vi "Drive Handling.vi"(1 "Reverse":bool, 2 "Straight":bool, 3 "Low Sensitivity":bool, 4 "Z":dbl, 5 "Y":dbl, 6 "X":dbl) -> (0 "Axes Magnitudes":cluster{"X":dbl, "Y":dbl, "Z":dbl})   [LabVIEW 2017, in "Huskie Swerve.lvlib"]
uses:
  Huskie Swerve.lvlib
panel:
  in  "Low Sensitivity x & y":dbl=1.7 format="%#_13g"
  in  "Low Sensitivity z":dbl=1.9 format="%#_13g"
  in  "Default Sensitivity x & y":dbl=1.4 format="%#_13g"
  in  "Default Sensitivity z":dbl=1.6 format="%#_13g"
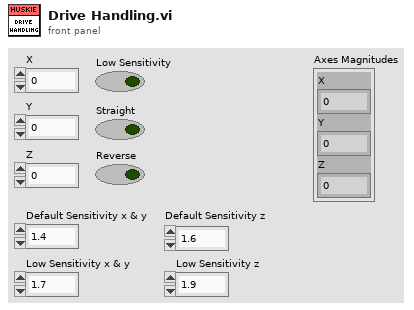
[diagram p1: front panel]
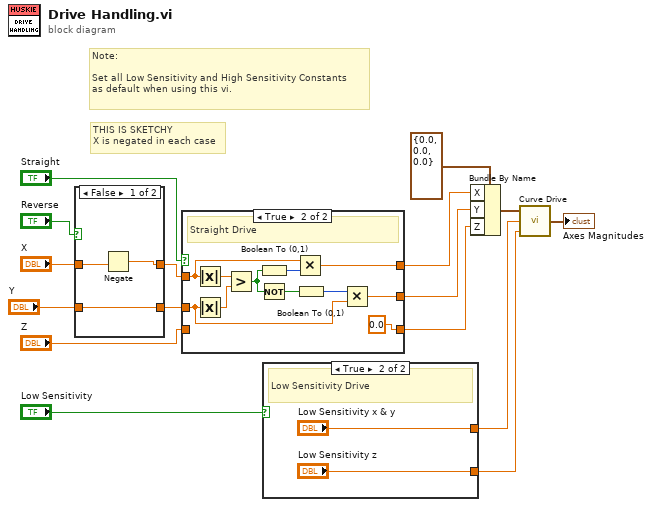
[diagram p0: block diagram]
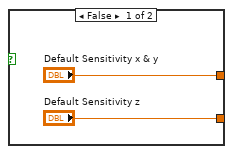
[diagram p2: hidden frame]
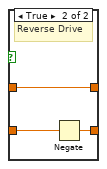
[diagram p4: hidden frame]
diagram:
  # "THIS IS SKETCHY\nX is negated in each case"
  # "Note: \n\nSet all Low Sensitivity and High Sensitivity Constants\nas default when using this vi."
  n1 = case shown="False" "Reverse" {
    tunnel: [w17 w20] -> w12
    tunnel: "X" -> [w18 w20]
    tunnel: [w19 w22] -> w13
    tunnel: "Y" -> [w19 w21]
    frame False {
      n2 = Negate(x=w18) -> (-x=w17:dbl)
    }
    frame True {
      # "Reverse Drive"
      n3 = Negate(x=w21) -> (-x=w22:dbl)
    }
  }
  n4 = case shown="True" "Straight" {
    tunnel: w12 -> [w25 w34]
    tunnel: w13 -> [w24 w29]
    tunnel: "Z" -> [w23 _]
    tunnel: [w25 w36] -> w5
    tunnel: [w23 0.0] -> w3
    tunnel: [w24 w35] -> w2
    frame False {
    }
    frame True {
      # "Straight Drive"
      n5 = Absolute Value(x=w34) -> (abs(x)=w28:dbl)
      n6 = Absolute Value(x=w29) -> (abs(x)=w27:dbl)
      n7 = Greater?(x=w28, y=w27) -> (0:w32:bool)
      n8 = Boolean To (0,1)(Boolean=w32) -> (0, 1=w33:i16)
      n9 = Not(x=w32) -> (.not. x?=w31:bool)
      n10 = Multiply(x=w34, y=w33) -> (x*y=w36:dbl)
      n11 = Boolean To (0,1)(Boolean=w31) -> (0, 1=w30:i16)
      n12 = Multiply(x=w30, y=w29) -> (x*y=w35:dbl)
    }
  }
  n13 = case shown="True" "Low Sensitivity" {
    tunnel: ["Default Sensitivity x & y" "Low Sensitivity x & y"] -> w8
    tunnel: ["Default Sensitivity z" "Low Sensitivity z"] -> w7
    frame False {
    }
    frame True {
      # "Low Sensitivity Drive"
    }
  }
  n14 = Bundle By Name(cluster=cluster{"X":dbl, "Y":dbl, "Z":dbl} {"X"=0.0, "Y"=0.0, "Z"=0.0} ("input cluster"), "X"=w5, "Y"=w2, "Z"=w3) -> (w4:cluster{"X":dbl, "Y":dbl, "Z":dbl})
  n15 = call "Curve Drive.vi"("z exponent"=w7, "x & y exponent"=w8, "Axes Magnitudes"=w4) -> ("Axes Magnitudes"=→"Axes Magnitudes":cluster{"X":dbl, "Y":dbl, "Z":dbl})
